vi "CreateParserFile.vi"(8 "error in (no error)":errorcluster, 11 "ArgumentParser in":refnum<class "ArgumentParser.lvclass">) -> (0 "error out":errorcluster, 3 "ArgumentParser out":refnum<class "ArgumentParser.lvclass">)   [LabVIEW 2022 SP3, in "ArgumentParser.lvlib" / "ArgumentParser.lvclass"]
uses:
  ArgumentParser.lvclass
  ArgumentParser.lvclass/ArgumentParser.ctl
  <vilib>/Utility/error.llb/Error Cluster From Error Code.vi
  <vilib>/ErrorRing/Error Ring.xnode
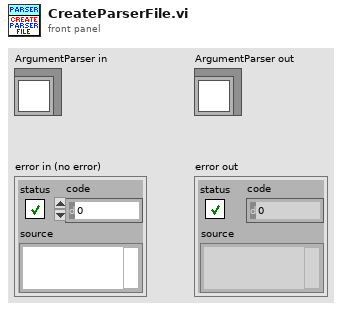
[diagram p1: front panel]
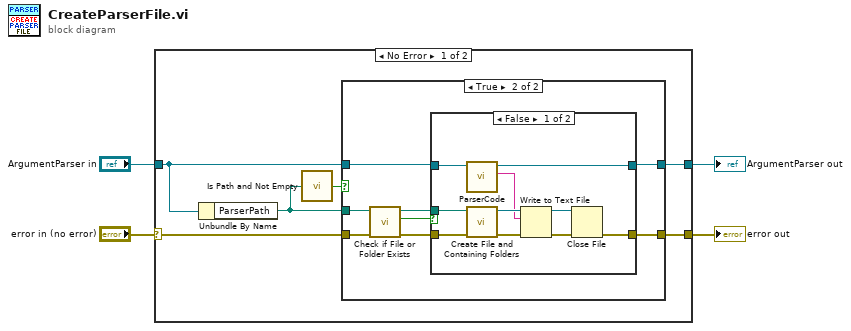
[diagram p0: block diagram]
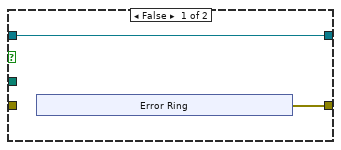
[diagram p2: hidden frame]
diagram:
  n1 = case shown="No Error" "error in (no error)" {
    selector: "error in (no error)" -> [w10 w39]
    tunnel: [w9 w39] -> w2
    tunnel: "ArgumentParser in" -> [w7 w38]
    tunnel: [w8 w38] -> w1
    frame No Error {
      n2 = Unbundle By Name(w7) -> ("ParserPath"=w6:path)
      n3 = call <vilib>:"Is Path and Not Empty.vi"("path"=w6) -> ("Is Path and Not Empty?"=w5:bool)  [unwired: 4 in]
      n4 = case shown="True" w5 {
        tunnel: w10 -> [_ w25]
        tunnel: [w11 w24] -> w9
        tunnel: [w12 w20] -> w8
        tunnel: w7 -> [w12 w19]
        tunnel: w6 -> [_ w18]
        frame False {
          n5 = xnode "Error Ring"() -> ("error out"=w11:errorcluster)
        }
        frame True {
          n6 = call <vilib>:"Check if File or Folder Exists.vi"("error in (no error)"=w25, "path"=w18) -> ("error out"=w23:errorcluster, "file or folder exists?"=w22:bool, "dup path"=w21:path)  [unwired: 7 in]
          n7 = case shown="False" w22 {
            tunnel: [w27 w37] -> w24
            tunnel: w23 -> [w34 w37]
            tunnel: w21 -> [w33 _]
            tunnel: [w29 w36] -> w20
            tunnel: w19 -> [w35 w36]
            frame False {
              n8 = call-dynamic "ParserCode.vi"("ArgumentParser in"=w35) -> ("ParserCode"=w28:string, "ArgumentParser out"=w29:refnum<class "ArgumentParser.lvclass">)  [unwired: 9 in]
              n9 = call <vilib>:"Create File and Containing Folders.vi"("error in (no error)"=w34, "file path"=w33) -> ("error out"=w32:errorcluster, "refnum out"=w30:refnum<file>)  [unwired: 8 in]
              n10 = Write to Text File(file (use dialog)=w30, text=w28, error in=w32) -> (refnum out=w26:refnum<file>, error out=w31:errorcluster)  [unwired: 1 in, 1 out]
              n11 = Close File(refnum=w26, error in=w31) -> (error out=w27:errorcluster)  [unwired: 1 out]
            }
            frame True {
            }
          }
        }
      }
    }
    frame Error {
    }
  }
  "error out" <- w2
  "ArgumentParser out" <- w1
